vi "Write Analog Output Channel.vi"(8 "error in (no error)":errorcluster, 10 "Analog Output Channel":tag="Dev1/ao1", 11 "Galvonometer in":refnum<class "Galvonometer.lvclass">) -> (0 "error out":errorcluster, 3 "Galvonometer out":refnum<class "Galvonometer.lvclass">)   [LabVIEW 2017, in "Galvonometer.lvclass"]
uses:
  Galvonometer.lvclass
  Galvonometer.lvclass/Galvonometer.ctl
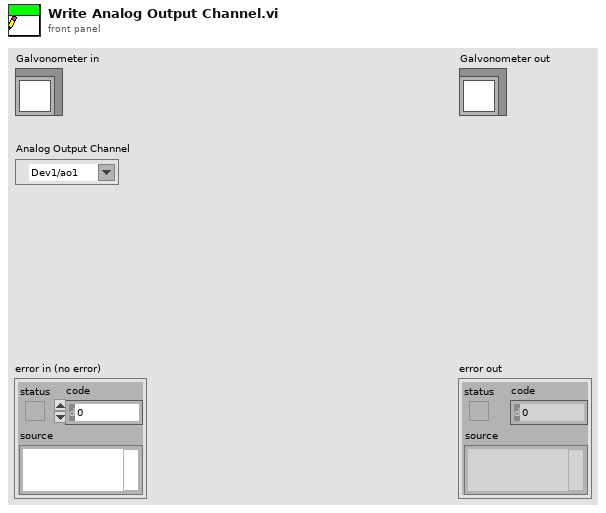
[diagram p1: front panel]
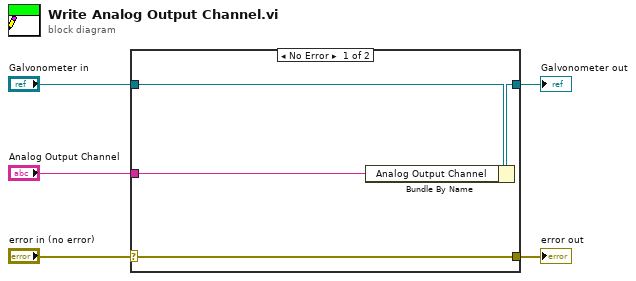
[diagram p0: block diagram]
diagram:
  n1 = case shown="No Error" "error in (no error)" {
    selector: "error in (no error)" -> [w9 w10]
    tunnel: [w9 w10] -> w4
    tunnel: [w7 w11] -> w2
    tunnel: "Galvonometer in" -> [w8 w11]
    tunnel: "Analog Output Channel" -> [w6 _]
    frame No Error {
      n2 = Bundle By Name(cluster=w8, "Analog Output Channel"=w6) -> (w7:refnum<class "Galvonometer.lvclass">)
    }
    frame Error {
    }
  }
  "error out" <- w4
  "Galvonometer out" <- w2
